vi "Read Scan Channels.vi"(8 "error in (no error)":errorcluster, 11 "LR-700 Driver in":refnum<class "LR-700 Driver.lvclass">) -> (0 "error out":errorcluster, 2 "Scan Channels":i32[](array[numeric]), 3 "LR-700 Driver out":refnum<class "LR-700 Driver.lvclass">)   [LabVIEW 2015, in "LR-700 Driver.lvclass"]
uses:
  LR-700 Driver.lvclass
  LR-700 Driver.lvclass/LR-700 Driver.ctl
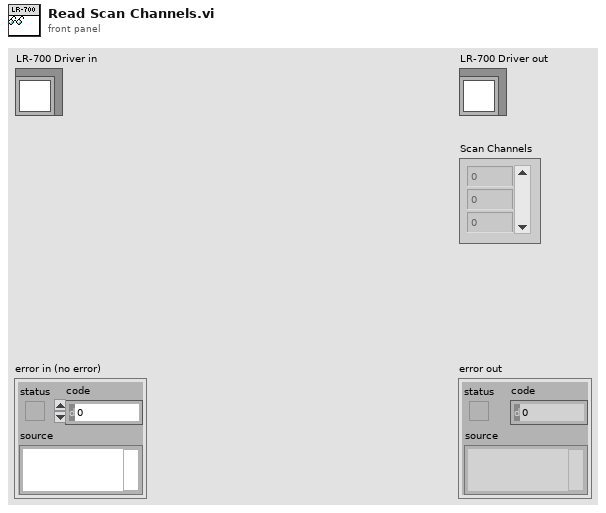
[diagram p1: front panel]
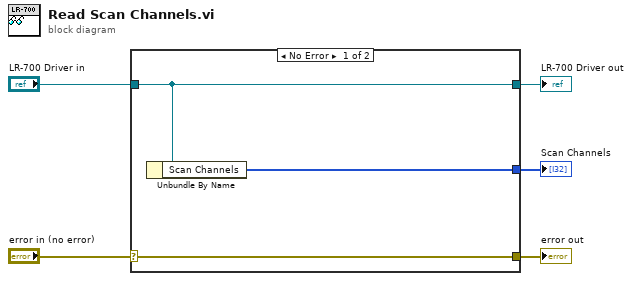
[diagram p0: block diagram]
diagram:
  n1 = case shown="No Error" "error in (no error)" {
    selector: "error in (no error)" -> [w8 w9]
    tunnel: [w8 w9] -> w4
    tunnel: [w7 w10] -> w2
    tunnel: "LR-700 Driver in" -> [w7 w10]
    tunnel: [w6 _] -> w1
    frame No Error {
      n2 = Unbundle By Name(w7) -> ("Scan Channels"=w6:i32[])
    }
    frame Error {
    }
  }
  "error out" <- w4
  "LR-700 Driver out" <- w2
  "Scan Channels" <- w1
